vi "FPGA_8tap 8bit_1_00.vi"() -> ()   [LabVIEW 2015]
uses:
  <vilib>/Platform/TimedLoop/XDataNode/timing_clust.ctl
  <vilib>/Platform/TimedLoop/XDataNode/nitl_modes.ctl
  <vilib>/Platform/TimedLoop/XDataNode/wakeup.ctl
  <vilib>/rvi/Emulation/niFpgaGetClockAttributes.vi
  <vilib>/rvi/Emulation/niFpgaSctlEmulationGetInTimedLoop.vi
  <vilib>/rvi/Emulation/niFpgaEmulationReportErrorSimple.vi
  <vilib>/rvi/Emulation/niFpgaProcessEmulError.vi
  <vilib>/rvi/Emulation/niFpgaCriticalErrorInLSC.vi
  <vilib>/rvi/eio/common/nirviEmuTemplateMethod_errors.vi
  Program Files (x86)/National Instruments/LabVIEW 2015/examples/Vision-RIO/Common/CL Data to Pixels/8 Tap 8-Bit.vi
  <vilib>/rvi/interface/RandomDataEmulation/nirviRandomDataMultiElementFPGAFIFO.vi
  <instcachedir>/0/nirviRandomDataMultiElementFPGAFIFO_8F99493546E24284B0D6A8E519C457F7.lvgen/nirviRandomDataMultiElementFPGAFIFO_8F99493546E24284B0D6A8E519C457F7_001.vi
  <vilib>/rvi/interface/RandomDataEmulation/niFpgaRandomDataHandleErrors.vi
  <vilib>/eio/EIONode/EIONode.xnode
  <vilib>/Platform/TimedLoop/XDataNode/XDataNode.xnode
  <vilib>/rvi/DataTransferAndStorage/Container/XNode/niFpgaContainer.xnode
  <vilib>/rvi/interface/RandomDataEmulation/nirviRandomDataFpgaMultiElementTemplate.vi
  <vilib>/Platform/TimedLoop/XDataNode/XDNodeRunTimeDep.lvlib
panel:
  in  "UART.Transmit":bool
  in  "UART.Tx Data":u8[](array[numeric])=[0, 0, 0, 0, 0, 0, 0, 0, 0, 0] format="%02x"
  in  "UART.Set Baud Rate":bool
  in  "UART.Byte Mode":bool=TRUE
  out "UART.Rx Ready":bool
  out "UART.Break Indicator":bool
  out "UART.Framing Error":bool
  out "UART.Overrun Error":bool
  out "UART.Tx Ready":bool
  out "UART.Rx Data":u8 format="%02x"
  in  "UART.Receive":bool
  in  "UART.Baud Rate":u8
  in  "Acq Control.Ignore DVAL":bool
  in  "Acq Control.Cancel Acq":bool
  in  "Acq Control.Acquire":bool
  out "Acq Status.Frames Acq'd":u32
  out "Acq Status.Lines Per Frame":u32
  out "Acq Status.Clocks Per Line":u32
  in  "Acq Control.Frames To Acq":u32
  out "Acq Status.Acq In Progress":bool
  in  "Acq Control.Line Scan Height":u32
  out "Acq Status.DMA Write Timeout":bool
  in  "Acq Control.Initialize":bool
  out "Acq Status.Initialized":bool
  in  "CL Config.DVAL Active High":bool=TRUE
  in  "CL Config.FVAL Active High":bool=TRUE
  in  "CL Config.LVAL Active High":bool=TRUE
  in  "CL Config.Spare Active High":bool=TRUE
  in  "CL Config.Line Scan":bool
  in  "CL Set Signal Mapping":u8
  in  "CL Set Configuration":u8
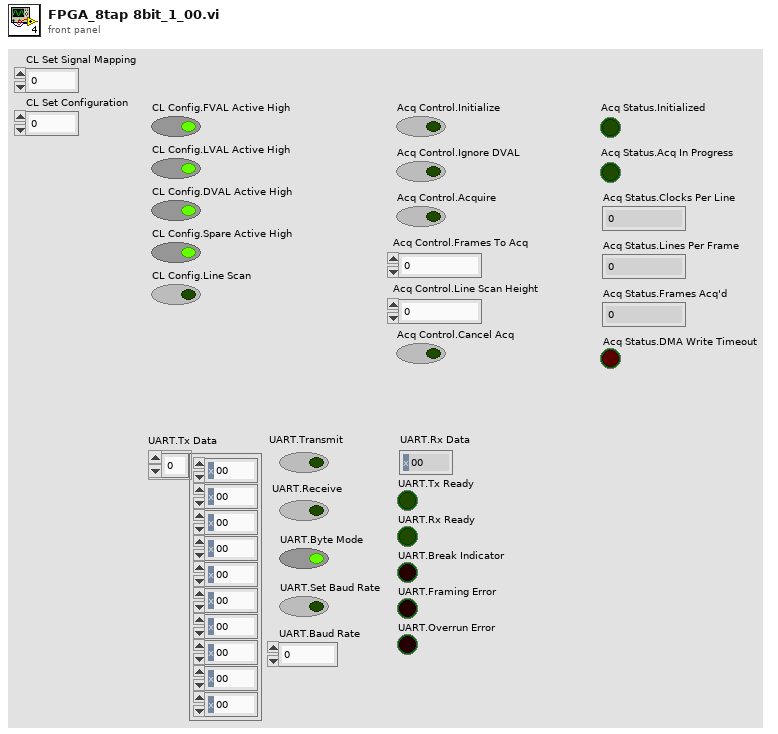
[diagram p1: front panel]
types:
  T1 = typedef "XDNodeRunTimeDep.lvlib/timing_clust.ctl" = cluster{"Expected End [f-1]":u64, "Actual End [f-1]":u64, "Finished Late? [f-1]":bool, "Expected End [i-1]":u64, "Actual End [i-1]":u64, "Finished Late? [i-1]":bool, "Expected Start [i]":u64, "Actual Start [i]":u64, "Expected Start [f]":u64, "Actual Start [f]":u64, "Source Name":string, "Structure Name":string, "Period":i64, "Deadline":i64, "Offset":i64, "Start":i64, "Priority":i32, "Timeout":i32, "Mode":T2, "Wakeup Reason":T3, "Error":errorcluster, "Source Type":string, "Secondary Source Type":string, "Global End Time":u64, "Global Start Time":u64, "Frame Duration":u64, "Iteration Duration":u64, "Assigned CPU":i32, "I/O Scan Engine Mode":u32}
  T2 = typedef "XDNodeRunTimeDep.lvlib/nitl_modes.ctl" = enum32{"No Change", "Process missed periods, maintain original phase", "Discard missed periods, maintain original phase", "Process missed periods, ignore original phase", "Discard missed periods, ignore original phase"}
  T3 = typedef "XDNodeRunTimeDep.lvlib/wakeup.ctl" = enum32{"Normal", "Aborted", "Asynchronous wakeup", "Timing source error", "Timed loop error", "Timeout"}
  T4 = cluster{"Enables Valid":bool, "Frame Valid":bool, "Line Valid":bool, "Data Valid":bool}
  T5 = cluster{"Pixel 0":u8, "Pixel 1":u8, "Pixel 2":u8, "Pixel 3":u8, "Pixel 4":u8, "Pixel 5":u8, "Pixel 6":u8, "Pixel 7":u8}
  T6 = cluster{"Tx Data":u8[], "Transmit":bool, "Receive":bool, "Byte Mode":bool, "Set Baud Rate":bool, "Baud Rate":u8}
  T7 = cluster{"Rx Data":u8, "Turn Off Transmit":bool, "Turn Off Receive":bool, "Turn Off Set Baud Rate":bool, "Tx Ready":bool, "Rx Ready":bool, "Break Indicator":bool, "Framing Error":bool, "Overrun Error":bool}
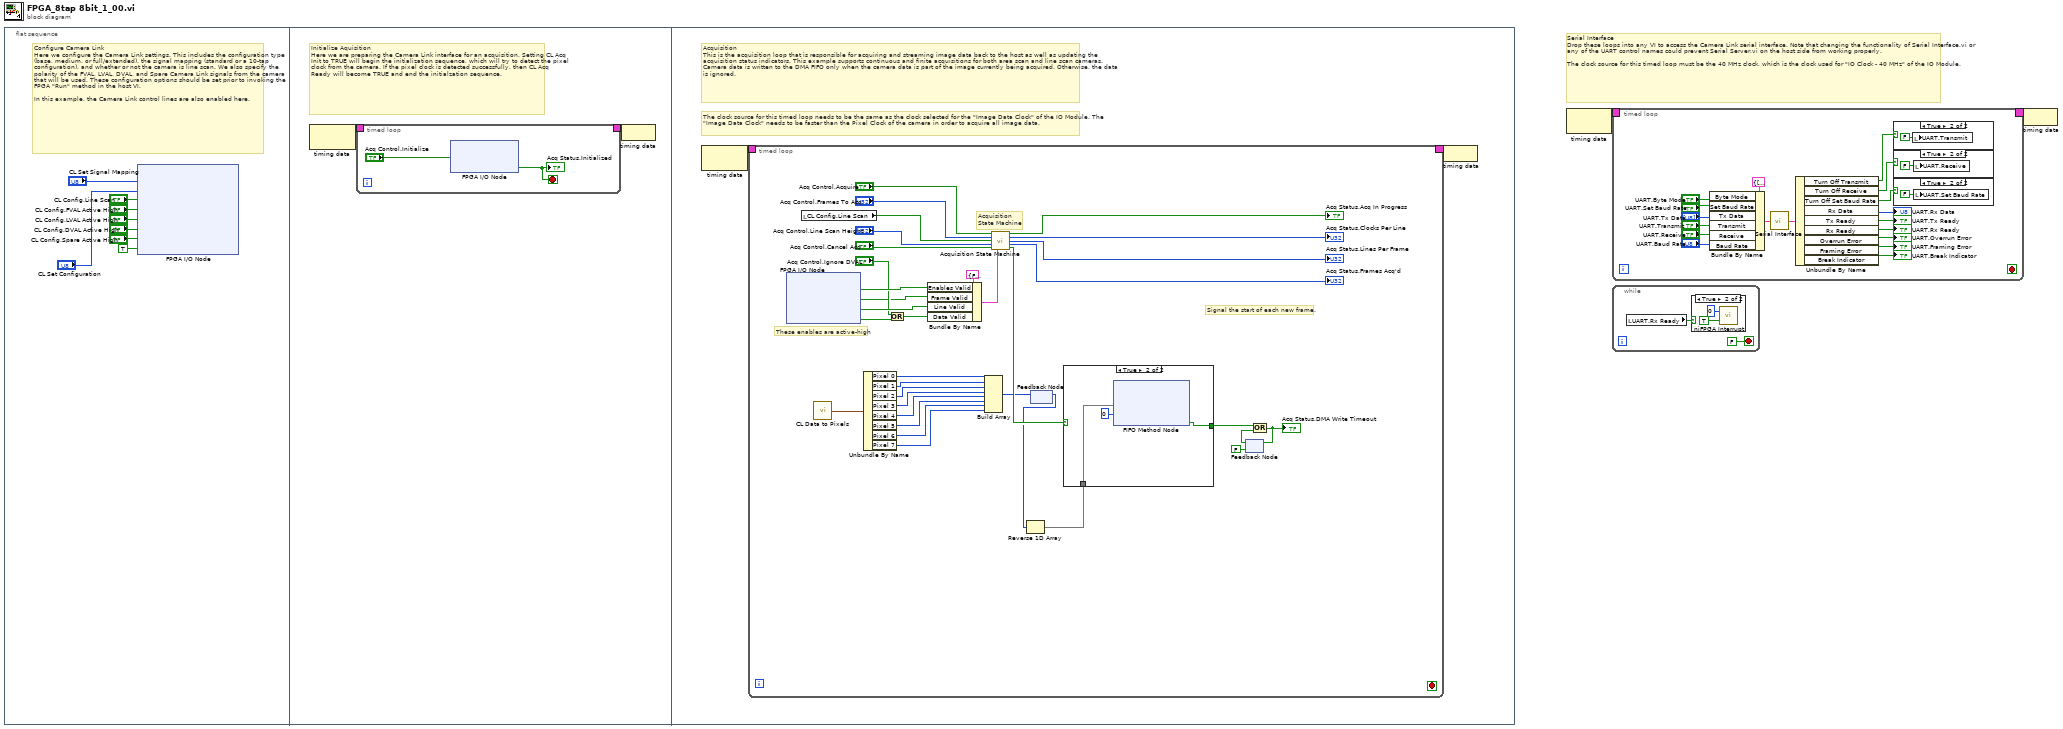
[diagram p0: block diagram]
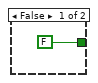
[diagram p6: hidden frame]
diagram:
  # "Serial Interface\nDrop these loops into any VI to access the Camera Link serial interface. Note that changing the functionality of Serial Interface.vi or any of the UART control names could prevent Serial Server.vi on the host side from working properly.\n\nThe clock source for this timed loop must be the 40 MHz clock, which is the clock used for \"IO Clock - 40 MHz\" of the IO Module."
  n1 = flat-sequence {
    frame #0 {
      # "Configure Camera Link\nHere we configure the Camera Link settings. This includes the configuration type (base, medium, or full/extended), the signal mapping (standard or a 10-tap configuration), and whether or not the camera is line scan. We also specify the polarity of the FVAL, LVAL, DVAL, and Spare Camera Link signals from the camera that will be used. These configuration options should be set prior to invoking the FPGA \"Run\" method in the host VI.\n\nIn this example, the Camera Link control lines are also enabled here."
      n2 = xnode "FPGA I/O Node"("CL Set Signal Mapping"="CL Set Signal Mapping", "CL Set Configuration"="CL Set Configuration", "CL Set Line Scan"="CL Config.Line Scan", "CL Set FVAL Active High"="CL Config.FVAL Active High", "CL Set LVAL Active High"="CL Config.LVAL Active High", "CL Set DVAL Active High"="CL Config.DVAL Active High", "CL Set Spare Active High"="CL Config.Spare Active High", "CL Control Enable"=TRUE ("IO Module\\CL Control Enable")) -> ()  [unwired: 8 in, 8 out]
    }
    frame #1 {
      # "Initialize Aquisition\nHere we are preparing the Camera Link interface for an acquisition. Setting CL Acq Init to TRUE will begin the initialization sequence, which will try to detect the pixel clock from the camera. If the pixel clock is detected successfully, then CL Acq Ready will become TRUE and end the initialzation sequence."
      n3 = node-c288() -> (w12:T1)  [unwired: 1 out]
      n4 = timed-loop {
        timing: w12 -> [_]
        timing-out: [_] -> w11
        stop <- w13 stop-if-true
        n5 = xnode "FPGA I/O Node"("CL Acq Init"="Acq Control.Initialize") -> ("CL Acq Ready"=w13:bool)  [unwired: 2 in, 2 out]
        "Acq Status.Initialized" <- w13
      }
      n6 = node-c288(w11) -> ()
    }
    frame #2 {
      # "The clock source for this timed loop needs to be the same as the clock selected for the \"Image Data Clock\" of the IO Module. The \"Image Data Clock\" needs to be faster than the Pixel Clock of the camera in order to acquire all image data."
      # "Acquisition\nThis is the acquisition loop that is responsible for acquiring and streaming image data back to the host as well as updating the acquisition status indicators. This example supports continuous and finite acquisitions for both area scan and line scan cameras. Camera data is written to the DMA FIFO only when the camera data is part of the image currently being acquired. Otherwise, the data is ignored."
      n7 = node-c288() -> (w20:T1)  [unwired: 1 in]
      n8 = timed-loop {
        timing: w20 -> [_]
        timing-out: [_] -> w19
        stop <- _ stop-if-true
        # "Signal the start of each new frame."
        # "These enables are active-high"
        # "Acquisition\nState Machine"
        n9 = xnode "FPGA I/O Node"() -> ("CL Output Valid"=w46:bool, "CL Frame Valid"=w37:bool, "CL Line Valid"=w45:bool, "CL Data Valid"=w42:bool)  [unwired: 4 in, 4 out]
        n10 = local read "CL Config.Line Scan"() -> (w39:bool)
        n11 = call-poly "CL Data to Pixels.vi"() -> ("Pixels"=w54:T5)  [unwired: 1 in]
        n12 = Unbundle By Name(w54) -> ("Pixel 0"=w36:u8, "Pixel 1"=w35:u8, "Pixel 2"=w34:u8, "Pixel 3"=w33:u8, "Pixel 4"=w32:u8, "Pixel 5"=w31:u8, "Pixel 6"=w30:u8, "Pixel 7"=w29:u8)
        n13 = Or(x="Acq Control.Ignore DVAL", y=w42) -> (x .or. y?=w41:bool)
        n14 = Bundle By Name(cluster=T4 {"Enables Valid"=FALSE, "Frame Valid"=FALSE, "Line Valid"=FALSE, "Data Valid"=FALSE} ("Enables"), "Enables Valid"=w46, "Frame Valid"=w37, "Line Valid"=w45, "Data Valid"=w41) -> (w44:T4)
        n15 = Build Array(w36, w35, w34, w33, w32, w31, w30, w29) -> (w23:u8[])
        n16 = call "Acquisition State Machine.vi"("Acquire"="Acq Control.Acquire", "Frames to Acquire"="Acq Control.Frames To Acq", "Line Scan"=w39, "Line Scan Height"="Acq Control.Line Scan Height", "Cancel Acq"="Acq Control.Cancel Acq", "Enables"=w44) -> ("Acq In Progress"=→"Acq Status.Acq In Progress":bool, "Num Clocks Per Line"=→"Acq Status.Clocks Per Line":u32, "Num Lines Per Frame"=→"Acq Status.Lines Per Frame":u32, "Num Frames Acq'd"=→"Acq Status.Frames Acq'd":u32, "Capture Cycle"=w24:bool)  [unwired: 4 in, 1 out]
        n17 = feedback-in #1(w23) -> ()
        n18 = feedback #1() -> (w21:u8[])  [unwired: 1 in]
        n19 = Reverse 1D Array(array=w21) -> (reversed array=w22:u8[])
        n20 = case shown="True" w24 {
          tunnel: [FALSE w57] -> w26
          tunnel: w22 -> [_ w56]
          frame False {
          }
          frame True {
            n21 = xnode ("FIFO Method Node")("Element"=w56, "Timeout"=0) -> ("Timed Out?"=w57:bool)  [unwired: 1 in, 1 out]
          }
        }
        n22 = feedback #2(FALSE) -> (w28:bool)
        n23 = Or(x=w26, y=w28) -> (x .or. y?=w25:bool)
        "Acq Status.DMA Write Timeout" <- w25
        n24 = feedback-in #2(w25) -> ()
      }
      n25 = node-c288(w19) -> ()
    }
  }
  n26 = node-c288() -> (w2:T1)  [unwired: 1 out]
  n27 = timed-loop {
    timing: w2 -> [_]
    timing-out: [_] -> w1
    stop <- _ stop-if-true
    n28 = Bundle By Name(cluster=T6 {"Tx Data"=[0, 0, 0, 0, 0, 0, 0, 0, 0, 0], "Transmit"=FALSE, "Receive"=FALSE, "Byte Mode"=TRUE, "Set Baud Rate"=FALSE, "Baud Rate"=0} ("UART Inputs"), "Byte Mode"="UART.Byte Mode", "Set Baud Rate"="UART.Set Baud Rate", "Tx Data"="UART.Tx Data", "Transmit"="UART.Transmit", "Receive"="UART.Receive", "Baud Rate"="UART.Baud Rate") -> (w63:T6)
    n29 = call "Serial Interface.vi"("UART Inputs"=w63) -> ("UART Outputs"=w75:T7)
    n30 = Unbundle By Name(w75) -> ("Turn Off Transmit"=w68:bool, "Turn Off Receive"=w69:bool, "Turn Off Set Baud Rate"=w65:bool, "Rx Data"=→"UART.Rx Data":u8, "Tx Ready"=→"UART.Tx Ready":bool, "Rx Ready"=→"UART.Rx Ready":bool, "Overrun Error"=→"UART.Overrun Error":bool, "Framing Error"=→"UART.Framing Error":bool, "Break Indicator"=→"UART.Break Indicator":bool)
    n31 = case shown="True" w68 {
      frame False {
      }
      frame True {
        n32 = local write "UART.Transmit"(FALSE ("UART.Transmit")) -> ()
      }
    }
    n33 = case shown="True" w69 {
      frame False {
      }
      frame True {
        n34 = local write "UART.Receive"(FALSE ("UART.Receive")) -> ()
      }
    }
    n35 = case shown="True" w65 {
      frame False {
      }
      frame True {
        n36 = local write "UART.Set Baud Rate"(FALSE ("UART.Receive")) -> ()
      }
    }
  }
  n37 = while {
    stop <- FALSE stop-if-true
    n38 = local read "UART.Rx Ready"() -> (w87:bool)
    n39 = case shown="True" w87 {
      frame False {
      }
      frame True {
        n40 = call <vilib>:"niFPGA Interrupt.vi"("Wait Until Cleared (F)"=TRUE ("Wait Until Cleared"), "IRQ Number (0)"=u8 0 ("IRQ Number")) -> ()  [unwired: 1 in]
      }
    }
  }
  n41 = node-c288(w1) -> ()
